vi "Switch_MotorP5_SoftFP.vi"(0 "reference in":refnum<class "Switch_MotorP5.lvclass">, 2 "Floating":bool, 5 "error in (no error)":errorcluster) -> (14 "reference out":refnum<class "Switch_MotorP5.lvclass">, 19 "error out":errorcluster)   [LabVIEW 2022 SP3, in "Switch_MotorP5.lvlib" / "Switch_MotorP5.lvclass"]
uses:
  Switch_MotorP5.lvclass
  Components/ViPER.lvlibp/ViPER.lvclass
  C:/Projects/Medulla/ViPER/Examples/Flux_Capacitor_Tester/Components/ViPER.lvlibp/ViPER.lvclass
panel:
  out "RPM":i32
  in  "Radio Buttons":T1(radio)=enum."M7"
  # "`"
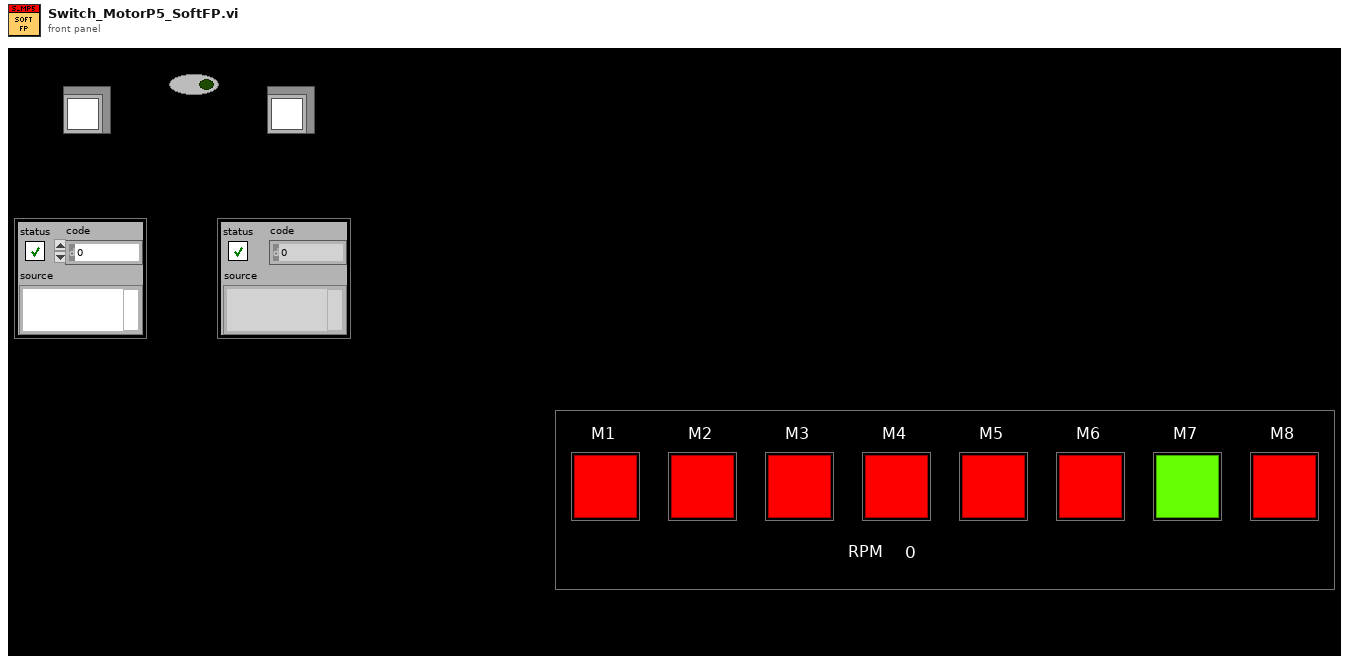
[diagram p1: front panel]
types:
  T1 = enum32{"M1", "M2", "M3", "M4", "M5", "M6", "M7", "M8"}
  T2 = enum32{"Invalid", "Standard", "Closed", "Hidden", "Minimized", "Maximized"}
  T3 = typedef "Switch_MotorP5.lvlib/Switch_MotorP5.lvclass/ObjectAttributes.ctl" = cluster{"Config":T4, "VISA":refnum<visa-resource-name>, "RPM":i32, "States":bool[], "UpdateEvent":refnum<user-event>, "Motor":enum32{"M1", "M2", "M3", "M4", "M5", "M6", "M7", "M8"}}
  T4 = typedef "Switch_MotorP5.lvlib/Switch_MotorP5.lvclass/Config.ctl" = cluster{"COM":refnum<visa-resource-name>, "SwitchMap":cluster{"Name":string, "Description":string, "Group":string, "IsGroup":bool, "Motor":enum32{"M1", "M2", "M3", "M4", "M5", "M6", "M7", "M8", "NA"}}[], "Sim":bool}
  T5 = cluster{"Name":string, "Description":string, "Group":string, "IsGroup":bool, "Motor":enum32{"M1", "M2", "M3", "M4", "M5", "M6", "M7", "M8", "NA"}}[]
  T6 = enum32{"M1", "M2", "M3", "M4", "M5", "M6", "M7", "M8", "NA"}
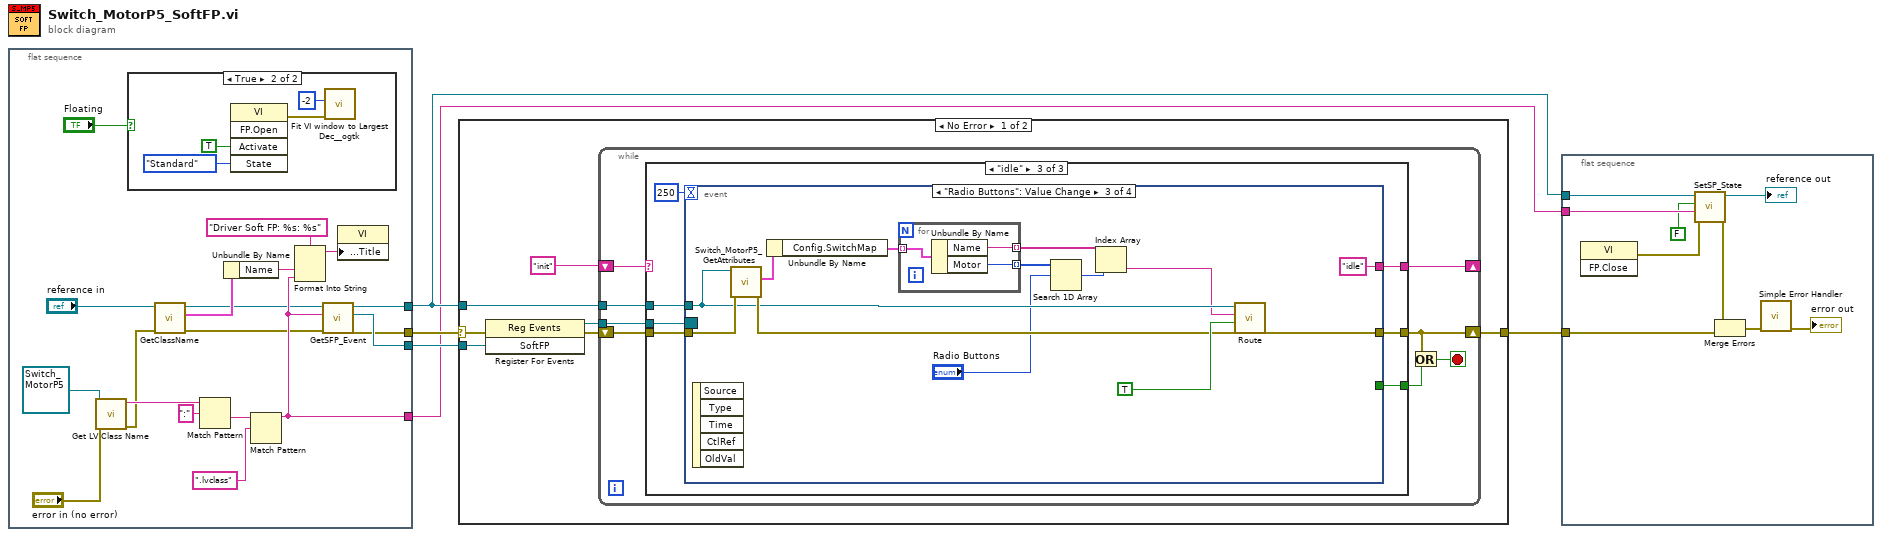
[diagram p0: block diagram]
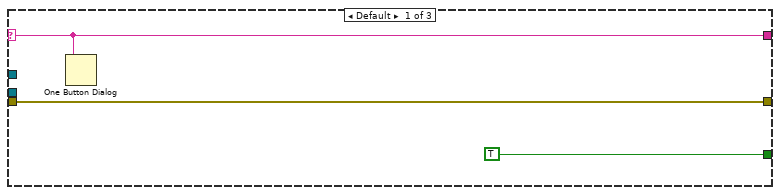
[diagram p3: hidden frame]
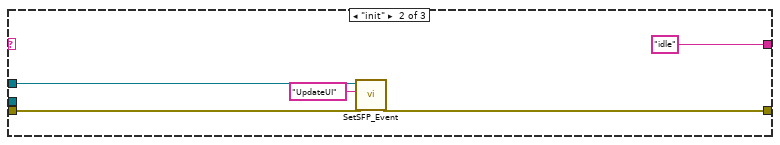
[diagram p4: hidden frame]
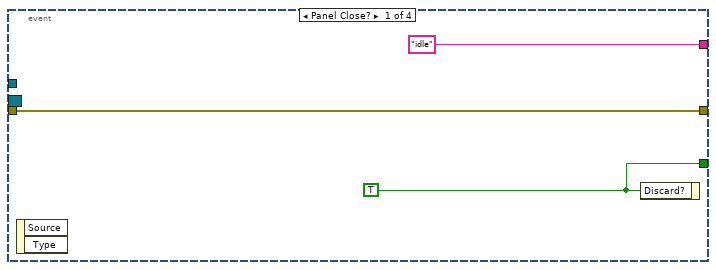
[diagram p5: hidden frame]
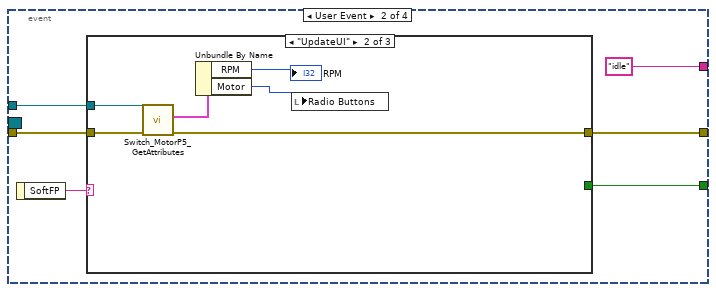
[diagram p6: hidden frame]
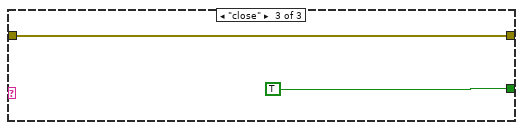
[diagram p8: hidden frame]
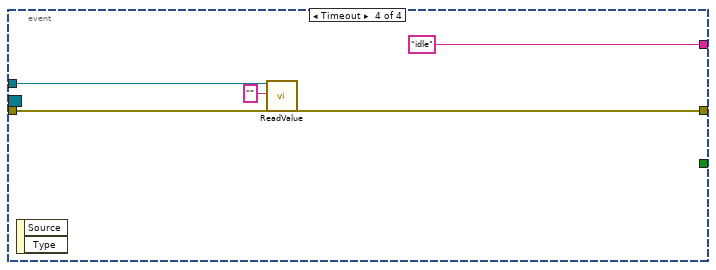
[diagram p9: hidden frame]
diagram:
  n1 = flat-sequence {
    tunnel: [w21] -> w5
    tunnel: [w20] -> w2
    tunnel: [w24] -> w3
    tunnel: [w12] -> w1
    frame #0 {
      n2 = call <vilib>:"Get LV Class Name.vi"("error in (no error)"="error in (no error)", "object"=refnum<class "Switch_MotorP5.lvclass"> refnum ("reference")) -> ("error out"=w11:errorcluster, "class name"=w17:string)  [unwired: 8 in]
      n3 = case shown="True" "Floating" {
        frame False {
        }
        frame True {
          n4 = invoke class="VI" method="FP.Open"("Activate"=TRUE ("Activate?"), "State"=T2."Standard") -> (error out=w25:errorcluster)  [unwired: 3 in, 4 out]
          n5 = call <userlib>:"Fit VI window to Largest Dec__ogtk.vi"("error in (no error)"=w25, "border spacing (2 px)"=-2) -> ()  [unwired: 4 in, 2 out]
        }
      }
      n6 = call "GetClassName.vi"("error in (no error)"=w11, "reference in"="reference in") -> ("error out"=w10:errorcluster, "Details"=w9:cluster{"Name":string, "Class":string}, "reference out"=w7:refnum<class "Switch_MotorP5.lvclass">)  [unwired: 7 in]
      n7 = Match Pattern(string=w17, regular expression=":") -> (after substring=w15:string)  [unwired: 1 in, 3 out]
      n8 = Unbundle By Name(w9) -> ("Name"=w19:string)
      n9 = Match Pattern(string=w15, regular expression=".lvclass") -> (before substring=w12:string)  [unwired: 1 in, 3 out]
      n10 = Format Into String(format string="Driver Soft FP: %s: %s", w19, w12) -> (resulting string=w23:string)  [unwired: 2 in, 1 out]
      n11 = call-dynamic "GetSFP_Event.vi"("error in (no error)"=w10, "Ancestor"=w12, "reference in"=w7) -> ("error out"=w21:errorcluster, "SoftFP"=w24:refnum<user-event>, "reference out"=w20:refnum<class "Switch_MotorP5.lvclass">)  [unwired: 6 in]
      n12 = property class="VI"("Front Panel.Title"=w23) -> ()  [unwired: 2 in, 2 out]
    }
  }
  n13 = case shown="No Error" w5 {
    selector: w5 -> [w33 w98]
    tunnel: [w29 w98] -> w4
    tunnel: w2 -> [w30 _]
    tunnel: w3 -> [w35 _]
    frame No Error {
      n14 = register-events(error in=w33, w35) -> (reference out=w34:refnum<event-registration>, error out=w32:errorcluster)  [unwired: 1 in]
      n15 = while {
        shift-right: [w40] -> w29
        shift-left: w32 -> [w43]
        tunnel: w34 -> [w42]
        tunnel: w30 -> [w41]
        shift-right: [w36] -> _
        shift-left: "init" -> [w37]
        stop <- w39 stop-if-true
        n16 = case shown="\"idle\"" w37 {
          selector: w37 -> [w44 _ _]
          tunnel: w43 -> [w45 w48 w58]
          tunnel: w42 -> [_ _ w57]
          tunnel: w41 -> [_ w47 w56]
          tunnel: [w45 w49 w55] -> w40
          tunnel: [TRUE ("Discard?") _ w54] -> w38
          tunnel: [w44 "idle" w53] -> w36
          frame Default {
            n17 = One Button Dialog(message=w44) -> ()  [unwired: 1 in, 1 out]
          }
          frame "init" {
            n18 = call-dynamic "SetSFP_Event.vi"("error in (no error)"=w48, "msg"="UpdateUI", "reference in"=w47) -> ("error out"=w49:errorcluster)  [unwired: 7 in, 1 out]
          }
          frame "idle" {
            n19 = event shown="[2] \"Radio Buttons\": Value Change" {
              selector: w57 -> [_ _ _ _]
              dyn-events: _ -> [_ _ _ _]
              timeout: 250 -> [_ _ _ _]
              tunnel: w58 -> [w61 w67 w85 w95]
              tunnel: [w61 w65 w89 w96] -> w55
              tunnel: [w60 w64 _ _] -> w54
              tunnel: w56 -> [_ w62 w84 w94]
              tunnel: ["idle" "idle" "idle" "idle"] -> w53
              event Panel Close? {
                w60 = TRUE ("Discard?")
                n20 = event-data() -> ()  [unwired: 1 in, 2 out]
                n21 = event-data("Discard?"=w60) -> ()  [unwired: 1 in, 1 out]
              }
              event User Event {
                n22 = event-data() -> ("SoftFP"=w66:string)  [unwired: 1 in]
                n23 = case shown="\"UpdateUI\"" w66 {
                  tunnel: w67 -> [w68 w73 w76]
                  tunnel: [w68 w74 w76] -> w65
                  tunnel: [_ _ TRUE ("Discard?")] -> w64
                  tunnel: w62 -> [_ w72 _]
                  frame Default {
                  }
                  frame "UpdateUI" {
                    n24 = call "Switch_MotorP5_GetAttributes.vi"("error in (no error)"=w73, "reference in"=w72) -> ("error out"=w74:errorcluster, "Data"=w71:T3)  [unwired: 6 in, 2 out]
                    n25 = Unbundle By Name(w71) -> ("RPM"=→"RPM":i32, "Motor"=w69:T1)
                    n26 = local write "Radio Buttons"(w69) -> ()
                  }
                  frame "close" {
                  }
                }
              }
              event "Radio Buttons": Value Change {
                n27 = event-data() -> ()  [unwired: 1 in, 5 out]
                n28 = call "Switch_MotorP5_GetAttributes.vi"("error in (no error)"=w85, "reference in"=w84) -> ("error out"=w86:errorcluster, "Data"=w83:T3)  [unwired: 6 in, 2 out]
                n29 = Unbundle By Name(w83) -> ("Config.SwitchMap"=w82:T5)
                n30 = for {
                  tunnel: w82 -> [w92] mode=indexing
                  tunnel: [w91] -> w78 mode=indexing
                  tunnel: [w90] -> w81 mode=indexing
                  n31 = Unbundle By Name(w92) -> ("Name"=w91:string, "Motor"=w90:T6)
                }
                n32 = Search 1D Array(1D array=w81, element="Radio Buttons") -> (index of element=w79:i32)  [unwired: 1 in]
                n33 = Index Array(array=w78, index=w79) -> (element=w77:string)
                n34 = call-dynamic "Route.vi"("error in (no error)"=w86, "Connect"=TRUE, "channel 1"=w77, "reference in"=w84) -> ("error out"=w89:errorcluster)  [unwired: 6 in, 1 out]
              }
              event Timeout {
                n35 = event-data() -> ()  [unwired: 1 in, 2 out]
                n36 = call-dynamic "ReadValue.vi"("reference in"=w94, "Name"="", "error in (no error)"=w95) -> ("error out"=w96:errorcluster)  [unwired: 14 in, 2 out]
              }
            }
          }
        }
        n37 = Or(x=w40, y=w38) -> (x .or. y?=w39:bool)
      }
    }
    frame Error {
    }
  }
  n38 = flat-sequence {
    tunnel: w4 -> [w105]
    tunnel: w2 -> [w100]
    tunnel: w1 -> [w102]
    frame #0 {
      n39 = invoke class="VI" method="FP.Close"() -> (error out=w104:errorcluster)  [unwired: 3 in, 2 out]
      n40 = call "SetSP_State.vi"("error in (no error)"=w104, "Ancestor"=w102, "SP Open"=FALSE, "reference in"=w100) -> ("error out"=w103:errorcluster, "reference out"=→"reference out":refnum<class "Switch_MotorP5.lvclass">)  [unwired: 6 in]
      n41 = Merge Errors(w103, w105) -> (w107:errorcluster)
      n42 = call <vilib>:"Simple Error Handler.vi"("error in (no error)"=w107) -> ("error out"=→"error out":errorcluster)  [unwired: 4 in, 4 out]
    }
  }
